vi "SM Create Event.vi"(8 "error in (no error)":errorcluster) -> (0 "error out":errorcluster, 3 "Req. Transition Event":refnum<user-event>)   [LabVIEW 2022 SP3, in "StateMachine.lvlib" / "HSE-State-Machine.lvlib"]
doc: "Creates the local user event used for requesting a transition.\n\n____\nHAMPEL SOFTWARE ENGINEERING v2.6.0 (2023-12-19 10:54)"
uses:
  HSE-State-Machine.lvlib
  SM Request Transition Argument--cluster.ctl
  SM_Transitions.ctl
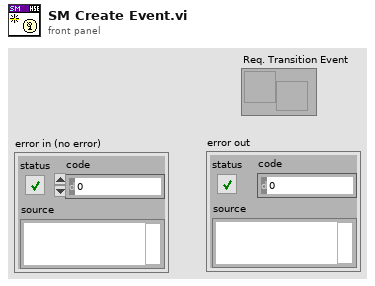
[diagram p1: front panel]
types:
  T1 = typedef "StateMachine.lvlib/HSE-State-Machine.lvlib/SM Request Transition Argument--cluster.ctl" = cluster{"Transition":T2, "Data":variant}
  T2 = typedef "StateMachine.lvlib/HSE-State-Machine.lvlib/SM_Transitions.ctl" = enum16{"No Transition", "Exception", "Reset", "Initialization finished", "Process started", "Trigger detected", "Exit"}
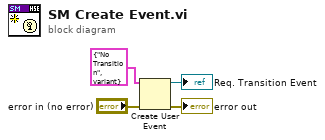
[diagram p0: block diagram]
diagram:
  n1 = Create User Event(user event datatype=T1 {"Transition"=enum."No Transition", "Data"=variant} ("Trigger HSE-SM Transition Argument"), error in="error in (no error)") -> (user event=→"Req. Transition Event":refnum<user-event>, error out=→"error out":errorcluster)
